vi "json Delete.vi"   [LabVIEW 2015, in "JSON Document.lvclass"]
uses:
  JSON Document.lvclass
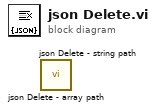
[diagram p0: block diagram]
diagram:
  n1 = call "json Delete - array path.vi"() -> ()  [unwired: 10 in, 2 out]
  n2 = call "json Delete - string path.vi"() -> ()  [unwired: 10 in, 2 out]
